vi "Create Version String.vi"(11 "Version":T1) -> (1 "Version info string":string, 3 "Version string":string)   [LabVIEW 2021, in "CIFLogs.lvlib"]
uses:
  CIFLogs.lvlib
  CIFCore/Common/Typedef/Version.ctl
  CIFCore/Common/CIFCoreCommon.lvlib
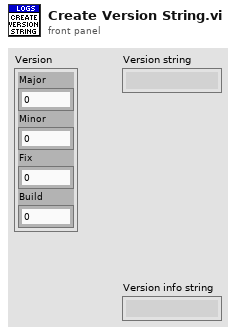
[diagram p1: front panel]
types:
  T1 = typedef "CIFCoreCommon.lvlib/Version.ctl" = cluster{"Major":i32, "Minor":i32, "Fix":i32, "Build":i32}
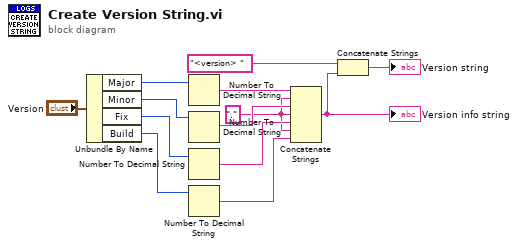
[diagram p0: block diagram]
diagram:
  w6 = "."
  n1 = Unbundle By Name("Version") -> ("Major"=w13:i32, "Minor"=w12:i32, "Fix"=w8:i32, "Build"=w9:i32)
  n2 = Number To Decimal String(number=w13) -> (decimal integer string=w11:string)  [unwired: 1 in]
  n3 = Number To Decimal String(number=w12) -> (decimal integer string=w10:string)  [unwired: 1 in]
  n4 = Number To Decimal String(number=w8) -> (decimal integer string=w7:string)  [unwired: 1 in]
  n5 = Number To Decimal String(number=w9) -> (decimal integer string=w5:string)  [unwired: 1 in]
  n6 = Concatenate Strings(w11, w6, w10, w6, w7, w6, w5) -> (w3:string)
  "Version info string" <- w3
  n7 = Concatenate Strings("<version> " ("string"), w3) -> (→"Version string":string)
